vi "TCPIP.vi"() -> ()   [LabVIEW 2014]
panel:
  out "concatenated string 2":string="TH-55ES630W,%71234567,4717523005417\r"
  out "bytes to read":i32
  out "Boolean":bool
  out "data out":string
  in  "Stop":bool
  in  "error in (no error)":errorcluster
  out "concatenated string":string
  in  "address":string="192.168.100.2"
  in  "data in":string="LON"
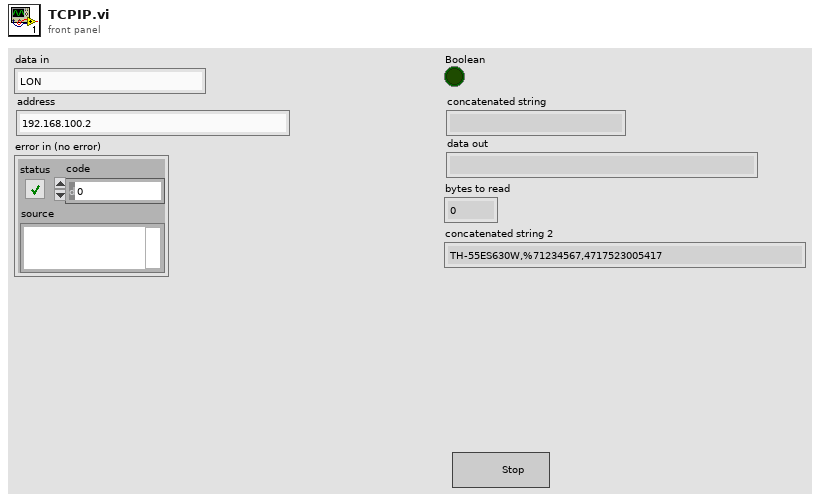
[diagram p1: front panel]
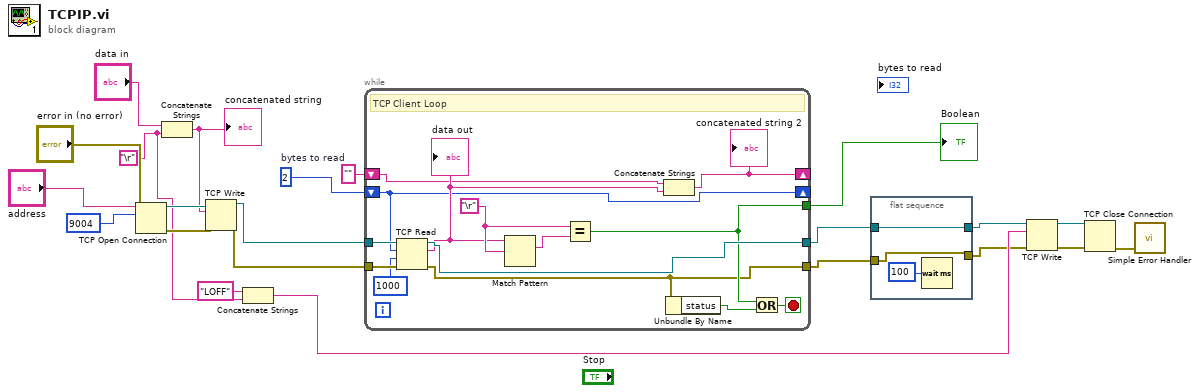
[diagram p0: block diagram]
diagram:
  w9 = 2  # bytes to read
  w15 = "\r"
  n1 = TCP Open Connection(address="address", remote port or service name=u16 9004, error in (no error)="error in (no error)") -> (connection ID=w22:refnum<k5>, error out=w21:errorcluster)  [unwired: 2 in]
  n2 = Concatenate Strings("data in", w15) -> (w18:string)
  "concatenated string" <- w18
  n3 = TCP Write(connection ID=w22, data in=w18, error in (no error)=w21) -> (connection ID out=w11:refnum<k5>, error out=w10:errorcluster)  [unwired: 1 in, 1 out]
  n4 = Concatenate Strings("LOFF" ("string"), w15) -> (w8:string)
  n5 = while {
    tunnel: w10 -> [w35]
    tunnel: w11 -> [w36]
    tunnel: [w30] -> w4
    tunnel: [w24] -> w2
    shift-right: [w25] -> _
    shift-left: w9 -> [w25]
    tunnel: [w29] -> w7
    shift-right: [w27] -> _
    shift-left: "" -> [w26]
    stop <- w34 stop-if-true
    w31 = "\r"
    # "TCP Client Loop"
    n6 = TCP Read(connection ID=w36, bytes to read=w25, error in (no error)=w35, 9:1000 ("timeout ms (25000)")) -> (connection ID out=w30:refnum<k5>, data out=w28:string, error out=w24:errorcluster)  [unwired: 1 in]
    "data out" <- w28
    n7 = Match Pattern(string=w28, regular expression=w31) -> (match substring=w32:string)  [unwired: 1 in, 3 out]
    n8 = Equal?(x=w31, y=w32) -> (x = y?=w29:bool)
    n9 = Concatenate Strings(w26, w28) -> (w27:string)
    "concatenated string 2" <- w27
    n10 = Unbundle By Name(w24) -> ("status"=w23:bool)
    n11 = Or(x=w29, y=w23) -> (x .or. y?=w34:bool)
  }
  "Boolean" <- w7
  n12 = flat-sequence {
    tunnel: w4 -> [w38]
    tunnel: [w38] -> w3
    tunnel: w2 -> [w37]
    tunnel: [w37] -> w1
    frame #0 {
      n13 = Wait (ms)(milliseconds to wait=u32 100) -> ()  [unwired: 1 out]
    }
  }
  n14 = TCP Write(connection ID=w3, data in=w8, error in (no error)=w1) -> (connection ID out=w12:refnum<k5>, error out=w13:errorcluster)  [unwired: 1 in, 1 out]
  n15 = TCP Close Connection(connection ID=w12, error in (no error)=w13) -> (error out=w5:errorcluster)  [unwired: 1 in, 1 out]
  n16 = call <vilib>:"Simple Error Handler.vi"("error in (no error)"=w5) -> ()  [unwired: 4 in, 5 out]
